vi "_LC Connect.vi"(7 "LC Type":T1) -> (0 "error out":errorcluster, 3 "Reply":string)   [LabVIEW 2015]
uses:
  Type/_LC Type.ctl
  Type/_LC Command.ctl
  Type/_Log Command.ctl
  _Global LC Driver.vi
panel:
  out "appended path":path
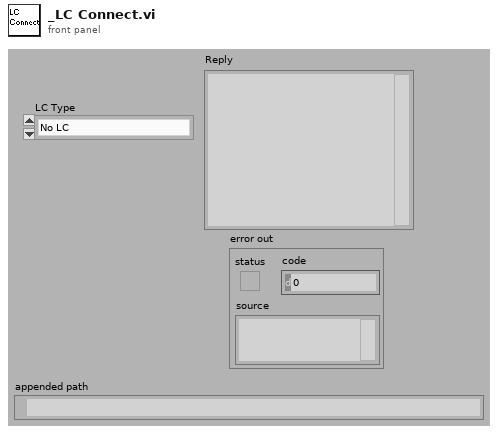
[diagram p1: front panel]
types:
  T1 = typedef "_LC Type.ctl" = enum16{"No LC", "Spark"}
  T2 = typedef "_LC Command.ctl" = enum16{"No Command", "Initialize", "Get Configuration", "Get Status", "Get LC Method Contents", "Oven OnOff", "Pump OnOFF", "Rinse Autosampler", "Run Sample", "Set EnvParameters", "Set Method", "Start Equilibration", "Stop Run", "Get LastError", "Clear Error", "Close"}
  T3 = typedef "_Log Command.ctl" = enum16{"No Command", "Open", "Read", "Write", "Close", "Check Size"}
  T4 = enum32{"Bad", "Idle", "Run top level", "Running"}
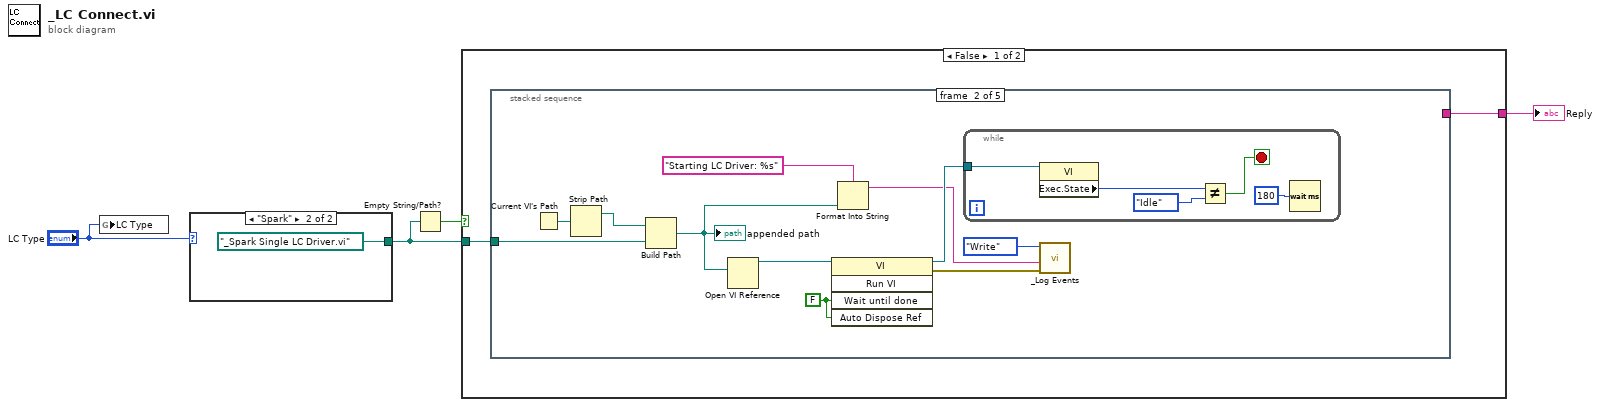
[diagram p0: block diagram]
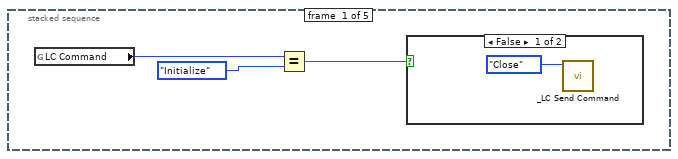
[diagram p2: hidden frame]
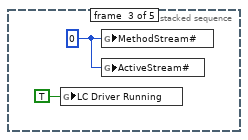
[diagram p4: hidden frame]
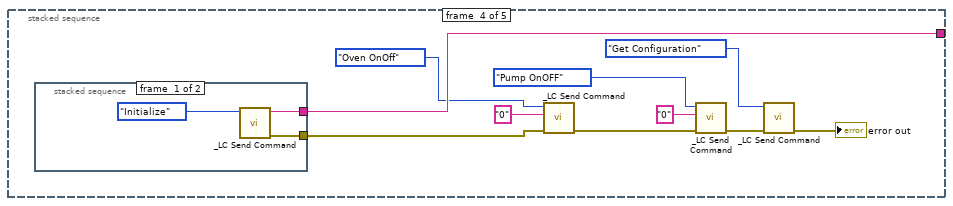
[diagram p5: hidden frame]
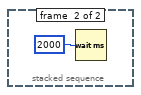
[diagram p6: hidden frame]
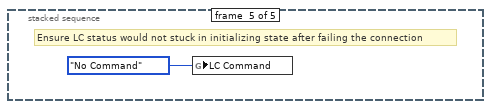
[diagram p7: hidden frame]
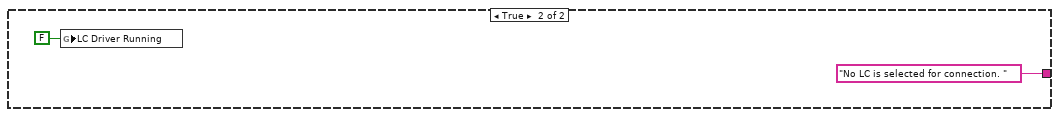
[diagram p8: hidden frame]
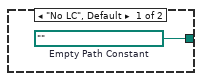
[diagram p9: hidden frame]
diagram:
  n1 = global write "_Global LC Driver.vi" "LC Type"("LC Type") -> ()
  n2 = case shown="\"Spark\"" "LC Type" {
    tunnel: [w5 path "_Spark Single LC Driver.vi" ("name or relative path")] -> w3
    frame "No LC", Default {
      w5 = path ""  # Empty Path Constant
    }
    frame "Spark" {
    }
  }
  n3 = Empty String/Path?(string/path=w3) -> (empty?=w4:bool)
  n4 = case shown="False" w4 {
    tunnel: w3 -> [w8 _]
    tunnel: [w7 "No LC is selected for connection. " ("Event")] -> w1
    frame False {
      n5 = stacked-sequence {
        tunnel: w8 -> [_ w19 _ _ _]
        tunnel: [_ _ _ w37 _] -> w7
        frame #0 {
          n6 = global read "_Global LC Driver.vi" "LC Command"() -> (w11:T2)
          n7 = Equal?(x=w11, y=_LC_Command."Initialize") -> (x = y?=w9:bool)
          n8 = case shown="False" w9 {
            frame False {
              n9 = call "_LC Send Command.vi"("Command"=_LC_Command."Close") -> ()  [unwired: 9 in, 2 out]
            }
            frame True {
              # "First time initializing"
            }
          }
        }
        frame #1 {
          w21 = FALSE ("Wait until done")
          n10 = Current VI's Path() -> (path=w23:path)
          n11 = Strip Path(path=w23) -> (stripped path=w22:path)  [unwired: 1 out]
          n12 = Build Path(base path=w22, name or relative path=w19) -> (appended path=w17:path)
          "appended path" <- w17
          n13 = Open VI Reference(vi path=w17) -> (vi reference=w20:refnum<vi>)  [unwired: 1 in, 5 out]
          n14 = invoke class="VI" method="Run VI"(reference=w20, "Wait until done"=w21, "Auto Dispose Ref"=w21) -> (reference out=w18:refnum<vi>, error out=w13:errorcluster)  [unwired: 2 in, 3 out]
          n15 = Format Into String(format string="Starting LC Driver: %s", w17) -> (resulting string=w15:string)  [unwired: 2 in, 1 out]
          n16 = while {
            tunnel: w18 -> [w28]
            stop <- w25 stop-if-true
            n17 = property class="VI"(reference=w28) -> ("Exec.State"=w27:T4)  [unwired: 1 in, 2 out]
            n18 = Not Equal?(x=w27, y=T4."Idle") -> (x != y?=w25:bool)
            n19 = Wait (ms)(milliseconds to wait=u32 180) -> ()  [unwired: 1 out]
          }
          n20 = call "_Log Events.vi"("error in (no error)"=w13, "Event"=w15, "Log Command"=_Log_Command."Write") -> ()  [unwired: 5 in, 2 out]
        }
        frame #2 {
          w29 = u8 0 ("MethodStream#")
          n21 = global write "_Global LC Driver.vi" "LC Driver Running"(TRUE ("LC Driver Running")) -> ()
          n22 = global write "_Global LC Driver.vi" "MethodStream#"(w29) -> ()
          n23 = global write "_Global LC Driver.vi" "ActiveStream#"(w29) -> ()
        }
        frame #3 {
          n24 = stacked-sequence {
            tunnel: [w42 _] -> w37
            tunnel: [w41 _] -> w31
            frame #0 {
              n25 = call "_LC Send Command.vi"("Command"=_LC_Command."Initialize") -> ("error out"=w41:errorcluster, "Reply"=w42:string)  [unwired: 9 in]
            }
            frame #1 {
              n26 = Wait (ms)(milliseconds to wait=u32 2000) -> ()  [unwired: 1 out]
            }
          }
          n27 = call "_LC Send Command.vi"("error in"=w31, "Parameter"="0" ("String In"), "Command"=_LC_Command."Oven OnOff") -> ("error out"=w34:errorcluster)  [unwired: 7 in, 1 out]
          n28 = call "_LC Send Command.vi"("error in"=w34, "Parameter"="0" ("String In"), "Command"=_LC_Command."Pump OnOFF") -> ("error out"=w35:errorcluster)  [unwired: 7 in, 1 out]
          n29 = call "_LC Send Command.vi"("error in"=w35, "Command"=_LC_Command."Get Configuration") -> ("error out"=→"error out":errorcluster)  [unwired: 8 in, 1 out]
        }
        frame #4 {
          # "Ensure LC status would not stuck in initializing state after failing the connection"
          n30 = global write "_Global LC Driver.vi" "LC Command"(_LC_Command."No Command" ("LC Command")) -> ()
        }
      }
    }
    frame True {
      n31 = global write "_Global LC Driver.vi" "LC Driver Running"(FALSE ("LC Driver Running")) -> ()
    }
  }
  "Reply" <- w1
